vi "Get Key Value (Text Reference).vi"(5 "Key name":string, 6 "Control reference":refnum<vi>, 7 "Section name":string, 8 "error in (no error)":errorcluster, 9 "Use LV Default? [F]":bool, 11 "Carya Config in":refnum<class "Carya Config.lvclass">) -> (0 "error out":errorcluster, 1 "Found?":bool, 2 "Value":string, 3 "Carya Config out":refnum<class "Carya Config.lvclass">)   [LabVIEW 2013, in "Carya Config.lvclass"]
doc: "Copyright 2018, Carya Automatisering, Wiebe Walstra."
uses:
  Carya Config.lvclass
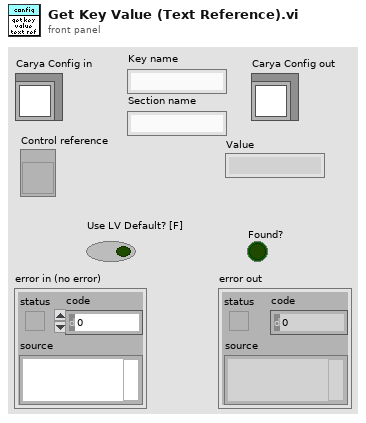
[diagram p1: front panel]
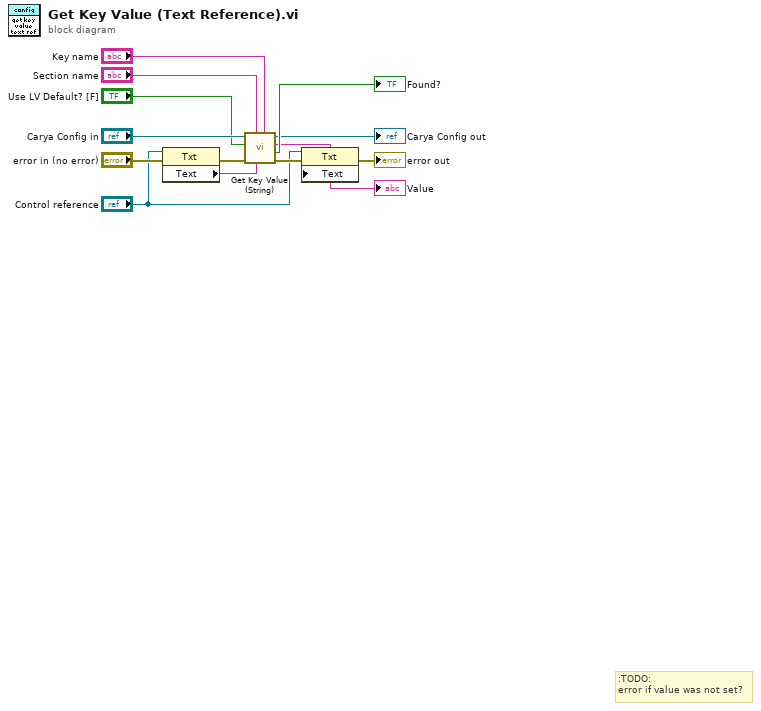
[diagram p0: block diagram]
diagram:
  # ":TODO:\nerror if value was not set?"
  n1 = property class="Txt"(reference="Control reference", error in="error in (no error)") -> (error out=w6:errorcluster, "Text"=w4:string)  [unwired: 1 out]
  n2 = call "Get Key Value (String).vi"("Key name"="Key name", "Default value"=w4, "Section name"="Section name", "error in (no error)"=w6, "Strip Whitespace? [T]"="Use LV Default? [F]", "Carya Config in"="Carya Config in") -> ("error out"=w12:errorcluster, "Found?"=→"Found?":bool, "Value"=w2:string, "Carya Config out"=→"Carya Config out":refnum<class "Carya Config.lvclass">)  [unwired: 2 in]
  "Value" <- w2
  n3 = property class="Txt"(reference="Control reference", error in=w12, "Text"=w2) -> (error out=→"error out":errorcluster)  [unwired: 1 out]
